vi "Main.vi"() -> ()   [LabVIEW 2013]
uses:
  <vilib>/Platform/TimedLoop/XDataNode/timing_clust.ctl
  <vilib>/Platform/TimedLoop/XDataNode/nitl_modes.ctl
  <vilib>/Platform/TimedLoop/XDataNode/wakeup.ctl
  <vilib>/myRIO/Common/Instrument Driver Framework/myRIO v1.0/DIO/vis/myRIO v1.1 Open DIO.vi
  <vilib>/myRIO/Common/Instrument Driver Framework/myRIO v1.0/DIO/vis/myRIO v1.0 Close DIO.vi
  <vilib>/myRIO/Common/Instrument Driver Framework/Utilities/vis/Validate Channels.vi
  <vilib>/myRIO/Common/Instrument Driver Framework/myRIO v1.0/DIO/vis/myRIO v1.0 Reserve DIO.vi
  <vilib>/myRIO/Common/Instrument Driver Framework/myRIO v1.0/DIO/vis/myRIO v1.0 Unreserve DIO.vi
  <vilib>/myRIO/Common/Instrument Driver Framework/myRIO v1.0/Resource Manager/vis/myRIO v1.0 Reserve Channel List.vi
  <vilib>/myRIO/Common/Instrument Driver Framework/myRIO v1.0/DIO/vis/myRIO v1.0 Build MUX Configuration DIO.vi
  <vilib>/myRIO/Common/Instrument Driver Framework/myRIO v1.0/Resource Manager/vis/myRIO v1.0 Unreserve Channel List.vi
  <vilib>/myRIO/Common/Instrument Driver Framework/myRIO v1.0/Resource Manager/vis/myRIO v1.0 Reserve Channel.vi
  <vilib>/myRIO/Common/Instrument Driver Framework/myRIO v1.0/Resource Manager/vis/myRIO v1.0 Unreserve Channel.vi
  <vilib>/myRIO/Common/Instrument Driver Framework/myRIO v1.0/Resource Manager/vis/myRIO v1.0 Create Configuration List.vi
  <vilib>/myRIO/Common/Instrument Driver Framework/myRIO v1.0/Resource Manager/vis/myRIO v1.0 Build Mutex Name.vi
  globals.vi
  <vilib>/myRIO/Common/Instrument Driver Framework/myRIO v1.0/myRIO v1.1 Open.vi
  <vilib>/Utility/VariantDataType/GetNumericInfo.vi
  <vilib>/Utility/error.llb/Error Cluster From Error Code.vi
  <vilib>/myRIO/Common/Instrument Driver Framework/Utilities/vis/IO Manager.vi
  <vilib>/myRIO/Common/Instrument Driver Framework/Utilities/vis/Configuration Manager.vi
  <vilib>/myRIO/Common/Instrument Driver Framework/myRIO v1.0/Resource Manager/vis/myRIO v1.0 Configure IO.vi
  <vilib>/myRIO/Common/Instrument Driver Framework/myRIO v1.0/myRIO v1.0 Close.vi
  <vilib>/myRIO/Common/Instrument Driver Framework/myRIO v1.0/DIO/vis/myRIO v1.0 Write DIO.vi
  <vilib>/myRIO/Common/Instrument Driver Framework/myRIO v1.0/DIO/vis/myRIO v1.0 Shutdown DIO.vi
  <vilib>/platform/TimedLoop/XDataNode/XDataNode.xnode
  <vilib>/myRIO/Instrument Drivers/Onboard IO/DIO/DIO.lvlib
  <vilib>/Platform/TimedLoop/XDataNode/XDNodeRunTimeDep.lvlib
panel:
  in  "Array":bool[][](array[boolean])
  in  "pattern loop time [ms]":u32(slide)=500 scale=10.0..1000.0
  in  "auto pattern":bool=TRUE
  out "green pattern":u64 format="%016x"
  out "red pattern":u64 format="%016x"
  in  "ESC":bool
  in  "green":bool[][](array[boolean])=[[FALSE, FALSE, FALSE, FALSE, FALSE, FALSE, FALSE, FALSE], [FALSE, FALSE, FALSE, FALSE, FALSE, FALSE, FALSE, FALSE], [FALSE, FALSE, FALSE, FALSE, FALSE, FALSE, FALSE, FALSE], [FALSE, FALSE, FALSE, FALSE, FALSE, FALSE, FALSE, FALSE], [FALSE, FALSE, FALSE, FALSE, FALSE, FALSE, FALSE, FALSE], [FALSE, FALSE, FALSE, FALSE, FALSE, FALSE, FALSE, FALSE], [FALSE, FALSE, FALSE, FALSE, FALSE, FALSE, FALSE, FALSE], [FALSE, FALSE, FALSE, FALSE, FALSE, FALSE, FALSE, FALSE]]
  in  "red":bool[][](array[boolean])=[[FALSE, FALSE, FALSE, FALSE, FALSE, FALSE, FALSE, FALSE], [FALSE, FALSE, FALSE, FALSE, FALSE, FALSE, FALSE, FALSE], [FALSE, FALSE, FALSE, FALSE, FALSE, FALSE, FALSE, FALSE], [FALSE, FALSE, FALSE, FALSE, FALSE, FALSE, FALSE, FALSE], [FALSE, FALSE, FALSE, FALSE, FALSE, FALSE, FALSE, FALSE], [FALSE, FALSE, FALSE, FALSE, FALSE, FALSE, FALSE, FALSE], [FALSE, FALSE, FALSE, FALSE, FALSE, FALSE, FALSE, FALSE], [FALSE, FALSE, FALSE, FALSE, FALSE, FALSE, FALSE, FALSE]]
  # "LED Matrix demo"
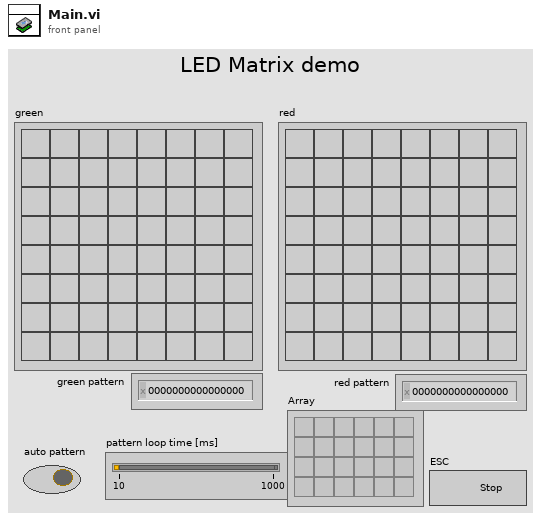
[diagram p1: front panel]
types:
  T1 = typedef "DIO.lvlib/DIO Reference.ctl" = cluster{"myRIO Reference":T2, "DIO Channels List":T6}
  T2 = typedef "myRIO Generic Hardware Reference.ctl" = cluster{"myRIO Model":T3, "myRIO Hardware Reference":T4}
  T3 = typedef "Hardware Version Enum.ctl" = enum16{"Unknown", "myRIO-1900", "myRIO-1950"}
  T4 = typedef "myRIO v1.0 Reference.ctl" = cluster{"Generic FPGA Reference":T5, "Allow multiple opens":bool}
  T5 = typedef "Generic FPGA Reference.ctl" = refnum<k20>
  T6 = typedef "DIO Channels List.ctl" = T7[]
  T7 = typedef "DIO Channels Enum.ctl" = enum16{"Not Connected", "C/DIO0", "C/DIO1", "C/DIO2", "C/DIO3", "C/DIO4", "C/DIO5", "C/DIO6", "C/DIO7", "A/DIO0", "A/DIO1", "A/DIO2", "A/DIO3", "A/DIO4", "A/DIO5", "A/DIO6", "A/DIO7", "A/DIO8", "A/DIO9", "A/DIO10", "A/DIO11", "A/DIO12", "A/DIO13", "A/DIO14", "A/DIO15", "B/DIO0", "B/DIO1", "B/DIO2", "B/DIO3", "B/DIO4", "B/DIO5", "B/DIO6", "B/DIO7", "B/DIO8", "B/DIO9", "B/DIO10", "B/DIO11", "B/DIO12", "B/DIO13", "B/DIO14", "B/DIO15", "LED0", "LED1", "LED2", "LED3", "Button0"}
  T8 = typedef "XDNodeRunTimeDep.lvlib/timing_clust.ctl" = cluster{"Expected End [f-1]":u64, "Actual End [f-1]":u64, "Finished Late? [f-1]":bool, "Expected End [i-1]":u64, "Actual End [i-1]":u64, "Finished Late? [i-1]":bool, "Expected Start [i]":u64, "Actual Start [i]":u64, "Expected Start [f]":u64, "Actual Start [f]":u64, "Source Name":string, "Structure Name":string, "Period":i64, "Deadline":i64, "Offset":i64, "Start":i64, "Priority":i32, "Timeout":i32, "Mode":T9, "Wakeup Reason":T10, "Error":errorcluster, "Source Type":string, "Secondary Source Type":string, "Global End Time":u64, "Global Start Time":u64, "Frame Duration":u64, "Iteration Duration":u64, "Assigned CPU":i32, "I/O Scan Engine Mode":u32}
  T9 = typedef "XDNodeRunTimeDep.lvlib/nitl_modes.ctl" = enum32{"No Change", "Process missed periods, maintain original phase", "Discard missed periods, maintain original phase", "Process missed periods, ignore original phase", "Discard missed periods, ignore original phase"}
  T10 = typedef "XDNodeRunTimeDep.lvlib/wakeup.ctl" = enum32{"Normal", "Aborted", "Asynchronous wakeup", "Timing source error", "Timed loop error", "Timeout"}
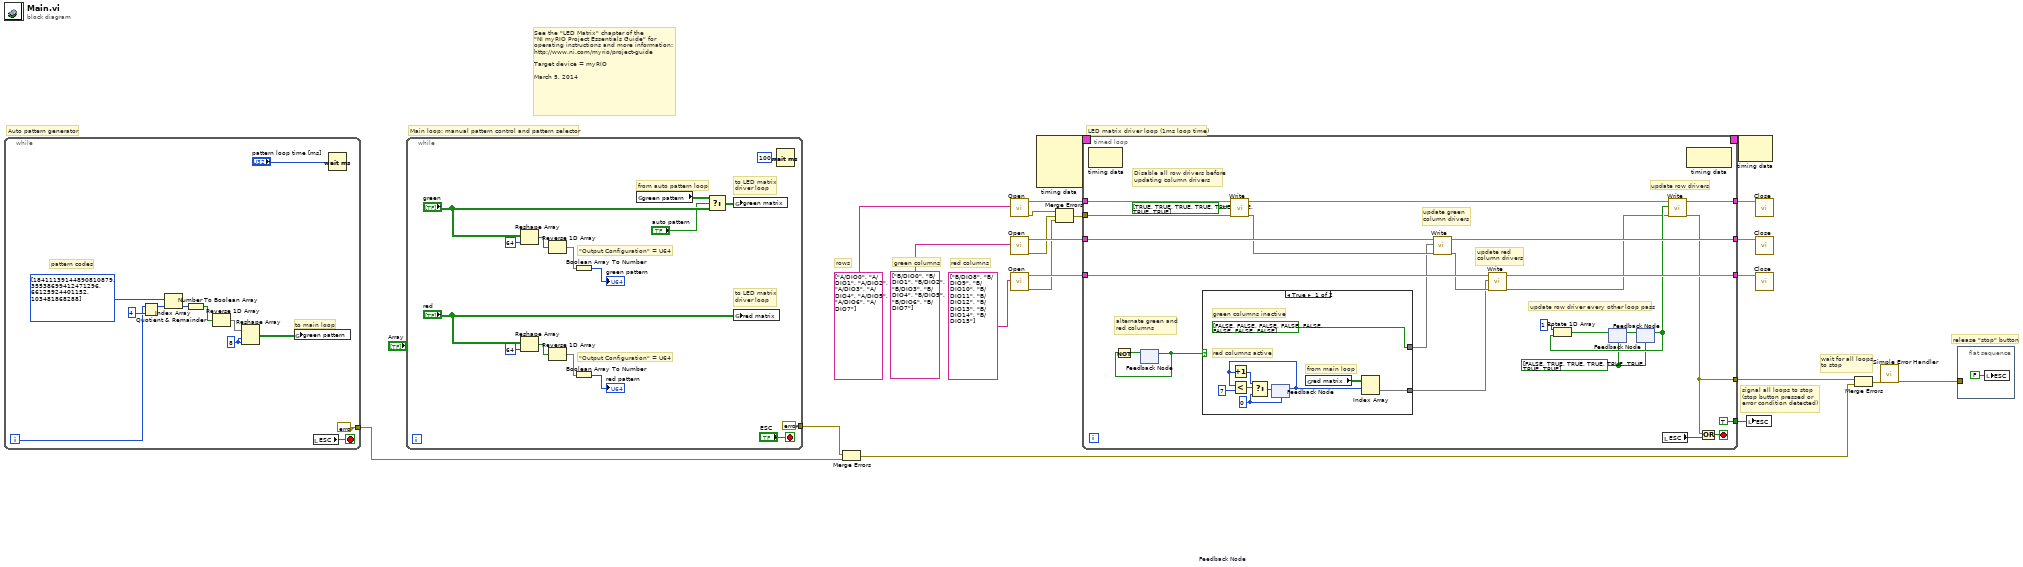
[diagram p0: block diagram]
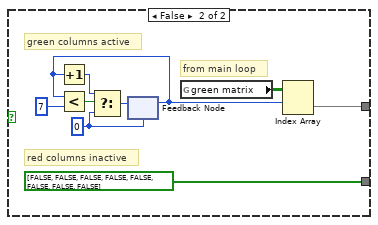
[diagram p2: hidden frame]
diagram:
  # "See the \"LED Matrix\" chapter of the\n\"NI myRIO Project Essentials Guide\" for\noperating instructions and more information: \nhttp://www.ni.com/myrio/project-guide\n\nTarget device = myRIO\n\nMarch 5, 2014"
  # "wait for all loops\nto stop"
  # "signal all loops to stop\n(stop button pressed or\nerror condition detected)"
  # "release \"stop\" button"
  # "Auto pattern generator"
  # "Main loop: manual pattern control and pattern selector"
  # "LED matrix driver loop (1ms loop time)"
  # "red columns"
  # "rows"
  # "green columns"
  n1 = while {
    tunnel: [errorcluster {"status"=FALSE, "code"=0, "source"=""} ("error constant")] -> w5
    i -> [w26]
    stop <- w24 stop-if-true
    w33 = 8 ("dimension size")
    # "to main loop"
    # "pattern codes"
    n2 = Quotient & Remainder(x=w26, y=4) -> (x-y*floor(x/y)=w29:i32)  [unwired: 1 out]
    n3 = Index Array "Index Array"(array=u64[] [18411139144890810879, 35538699412471296, 66125924401152, 103481868288], index=w29) -> (element=w30:u64)
    n4 = Number To Boolean Array(number=w30) -> (Boolean array=w31:bool[])
    n5 = Reverse 1D Array(array=w31) -> (reversed array=w32:bool[])
    n6 = Reshape Array "Reshape Array"(w32, w33, w33) -> (w25:bool[][])
    n7 = global write "globals.vi" "green pattern"(w25) -> ()
    n8 = local read "ESC"() -> (w24:bool)
    n9 = Wait (ms)(milliseconds to wait="pattern loop time [ms]") -> ()  [unwired: 1 out]
  }
  n10 = while {
    tunnel: [errorcluster {"status"=FALSE, "code"=0, "source"=""} ("error constant")] -> w4
    stop <- "ESC" stop-if-true
    # "from auto pattern loop"
    # "to LED matrix\ndriver loop"
    # "to LED matrix\ndriver loop"
    # "\"Output Configuration\" = U64"
    # "\"Output Configuration\" = U64"
    n11 = Reshape Array "Reshape Array"("green", 64 ("dimension size")) -> (w44:bool[])
    n12 = Reshape Array "Reshape Array"("red", 64 ("dimension size")) -> (w47:bool[])
    n13 = Reverse 1D Array(array=w44) -> (reversed array=w45:bool[])
    n14 = Reverse 1D Array(array=w47) -> (reversed array=w46:bool[])
    n15 = Boolean Array To Number(Boolean array=w45) -> (number=→"green pattern":u64)
    n16 = Boolean Array To Number(Boolean array=w46) -> (number=→"red pattern":u64)
    n17 = global read "globals.vi" "green pattern"() -> (w38:bool[][])
    n18 = Select(t=w38, s="auto pattern", f="green") -> (s? t:f=w35:bool[][])
    n19 = global write "globals.vi" "green matrix"(w35) -> ()
    n20 = global write "globals.vi" "red matrix"("red") -> ()
    n21 = Wait (ms)(milliseconds to wait=u32 100) -> ()  [unwired: 1 out]
  }
  n22 = Merge Errors(w4, w5) -> (w1:errorcluster)
  n23 = call <vilib>:"Open.vi"("Channel Names"=tag[] ["A/DIO0", "A/DIO1", "A/DIO2", "A/DIO3", "A/DIO4", "A/DIO5", "A/DIO6", "A/DIO7"]) -> ("error out"=w9:errorcluster, "DIO Ref Out"=w17:T1)  [unwired: 9 in]
  n24 = call <vilib>:"Open.vi"("Channel Names"=tag[] ["B/DIO0", "B/DIO1", "B/DIO2", "B/DIO3", "B/DIO4", "B/DIO5", "B/DIO6", "B/DIO7"]) -> ("error out"=w10:errorcluster, "DIO Ref Out"=w21:T1)  [unwired: 9 in]
  n25 = call <vilib>:"Open.vi"("Channel Names"=tag[] ["B/DIO8", "B/DIO9", "B/DIO10", "B/DIO11", "B/DIO12", "B/DIO13", "B/DIO14", "B/DIO15"]) -> ("error out"=w11:errorcluster, "DIO Ref Out"=w22:T1)  [unwired: 9 in]
  n26 = node-c288() -> (w13:T8)  [unwired: 4 in]
  n27 = Merge Errors(w9, w10, w11) -> (w8:errorcluster)
  n28 = timed-loop {
    tunnel: w22 -> [w63]
    tunnel: w21 -> [w64]
    tunnel: [w73] -> w20
    tunnel: [w72] -> w19
    tunnel: w17 -> [w68]
    tunnel: [w71] -> w16
    timing: w13 -> [_]
    timing-out: [_] -> w12
    tunnel: w8 -> [w65]
    tunnel: [w51] -> w3
    tunnel: [TRUE] -> w6
    stop <- w53 stop-if-true
    w57 = bool[] [FALSE, TRUE, TRUE, TRUE, TRUE, TRUE, TRUE, TRUE]
    # "update row drivers"
    # "update red\ncolumn drivers"
    # "update green\ncolumn drivers"
    # "Disable all row drivers before\nupdating column drivers"
    # "alternate green and\nred columns"
    # "update row driver every other loop pass"
    n29 = node-c288() -> ()  [unwired: 1 in, 1 out]
    n30 = feedback #1 "Feedback Node"() -> (w58:bool)  [unwired: 1 in]
    n31 = Not(x=w58) -> (.not. x?=w59:bool)
    n32 = feedback-in #1(w59) -> ()
    n33 = case shown="True" w58 {
      tunnel: [bool[] [FALSE, FALSE, FALSE, FALSE, FALSE, FALSE, FALSE, FALSE] w86] -> w56
      tunnel: [w78 bool[] [FALSE, FALSE, FALSE, FALSE, FALSE, FALSE, FALSE, FALSE]] -> w55
      frame True {
        w84 = 0 ("f")
        # "from main loop"
        # "green columns inactive"
        # "red columns active"
        n34 = feedback #2(w84) -> (w79:i32)
        n35 = Increment(x=w79) -> (x+1=w83:i32)
        n36 = Less?(x=w79, y=7) -> (x < y?=w82:bool)
        n37 = Select(t=w83, s=w82, f=w84) -> (s? t:f=w80:i32)
        n38 = feedback-in #2(w80) -> ()
        n39 = global read "globals.vi" "red matrix"() -> (w76:bool[][])
        n40 = Index Array "Index Array"(array=w76, index (row)=w79) -> (element=w78:bool[])  [unwired: 1 in]
      }
      frame False {
        w93 = 0 ("f")
        # "from main loop"
        # "red columns inactive"
        # "green columns active"
        n41 = feedback #3(w93) -> (w88:i32)
        n42 = Increment(x=w88) -> (x+1=w92:i32)
        n43 = Less?(x=w88, y=7) -> (x < y?=w91:bool)
        n44 = Select(t=w92, s=w91, f=w93) -> (s? t:f=w89:i32)
        n45 = feedback-in #3(w89) -> ()
        n46 = global read "globals.vi" "green matrix"() -> (w85:bool[][])
        n47 = Index Array "Index Array"(array=w85, index (row)=w88) -> (element=w86:bool[])  [unwired: 1 in]
      }
    }
    n48 = call <vilib>:"Write.vi"("error in (no error)"=w65, "Values"=bool[] [TRUE, TRUE, TRUE, TRUE, TRUE, TRUE, TRUE, TRUE], "DIO Ref In"=w68) -> ("error out"=w62:errorcluster, "DIO Ref Out"=w67:T1)  [unwired: 6 in]
    n49 = call <vilib>:"Write.vi"("error in (no error)"=w62, "Values"=w56, "DIO Ref In"=w64) -> ("error out"=w61:errorcluster, "DIO Ref Out"=w73:T1)  [unwired: 6 in]
    n50 = call <vilib>:"Write.vi"("error in (no error)"=w61, "Values"=w55, "DIO Ref In"=w63) -> ("error out"=w60:errorcluster, "DIO Ref Out"=w72:T1)  [unwired: 6 in]
    n51 = feedback #4(w57) -> (w70:bool[])
    n52 = feedback #5(w57) -> (w69:bool[])
    n53 = Rotate 1D Array(1:w69, 2:1 ("n")) -> (0:w74:bool[])
    n54 = feedback-in #4(w74) -> ()
    n55 = feedback-in #5(w70) -> ()
    n56 = local read "ESC"() -> (w54:bool)
    n57 = call <vilib>:"Write.vi"("error in (no error)"=w60, "Values"=w69, "DIO Ref In"=w67) -> ("error out"=w51:errorcluster, "DIO Ref Out"=w71:T1)  [unwired: 6 in]
    n58 = node-c288() -> ()  [unwired: 1 in, 1 out]
    n59 = Or(x=w51, y=w54) -> (x .or. y?=w53:bool)
  }
  n60 = node-c288(w12) -> ()  [unwired: 1 out]
  n61 = local write "ESC"(w6) -> ()
  n62 = call <vilib>:"Close.vi"("DIO Ref In"=w16) -> ()  [unwired: 10 in, 1 out]
  n63 = call <vilib>:"Close.vi"("DIO Ref In"=w20) -> ()  [unwired: 10 in, 1 out]
  n64 = call <vilib>:"Close.vi"("DIO Ref In"=w19) -> ()  [unwired: 10 in, 1 out]
  n65 = Merge Errors(w3, w1) -> (w2:errorcluster)
  n66 = call <vilib>:"Simple Error Handler.vi"("error in (no error)"=w2) -> ("error out"=w7:errorcluster)  [unwired: 4 in, 4 out]
  n67 = flat-sequence {
    tunnel: w7 -> [_]
    frame #0 {
      n68 = local write "ESC"(FALSE ("ESC")) -> ()
    }
  }
